vi "Close.vi"(8 "error in (no error)":errorcluster, 11 "E5071C in":refnum<class "E5071C.lvclass">) -> (0 "error out":errorcluster, 3 "E5071C out":refnum<class "E5071C.lvclass">)   [LabVIEW 2020, in "E5071C.lvlib" / "E5071C.lvclass"]
uses:
  E5071C.lvclass
  E5071C.lvclass/E5071C.ctl
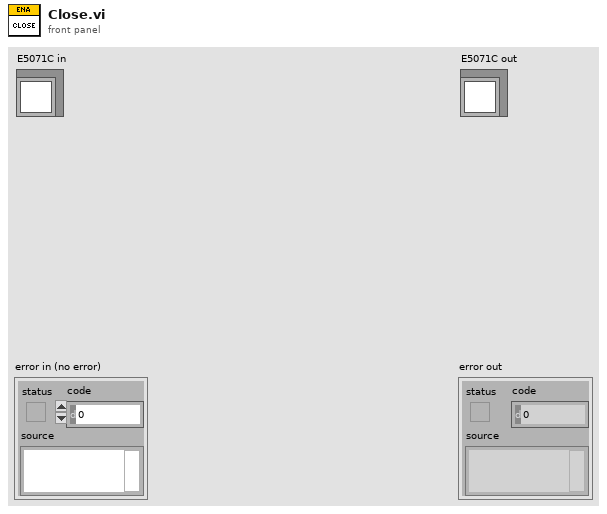
[diagram p1: front panel]
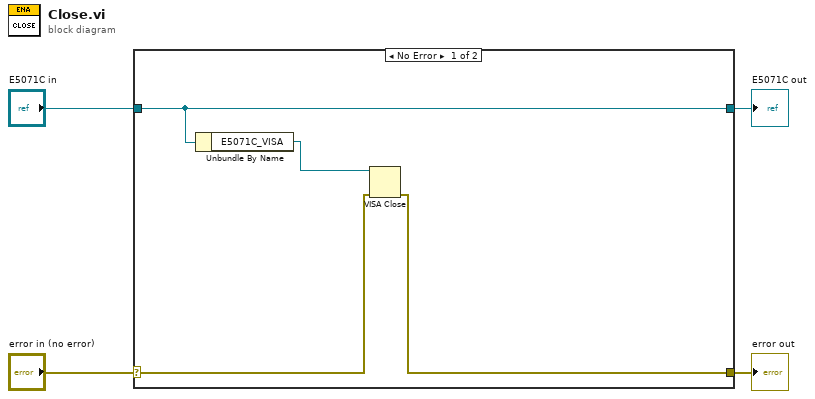
[diagram p0: block diagram]
diagram:
  n1 = case shown="No Error" "error in (no error)" {
    selector: "error in (no error)" -> [w6 w10]
    tunnel: [w5 w10] -> w3
    tunnel: [w8 w9] -> w1
    tunnel: "E5071C in" -> [w8 w9]
    frame No Error {
      n2 = Unbundle By Name(w8) -> ("E5071C_VISA"=w7:refnum<visa-resource-name>)
      n3 = VISA Close(VISA resource name=w7, error in (no error)=w6) -> (error out=w5:errorcluster)
    }
    frame Error {
    }
  }
  "error out" <- w3
  "E5071C out" <- w1
